vi "SetMode.vi"(0 "VISA resource name":refnum<visa-resource-name>, 5 "Combo Box":string(combo), 11 "error in (no error)":errorcluster) -> (4 "VISA resource name out":refnum<visa-resource-name>, 15 "error out":errorcluster)   [LabVIEW 2024, in "EFmeter.lvlib"]
uses:
  EFmeter.lvlib
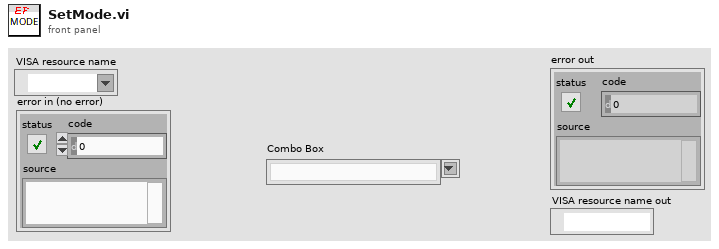
[diagram p1: front panel]
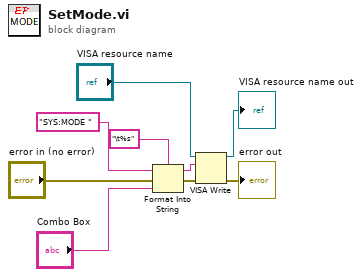
[diagram p0: block diagram]
diagram:
  n1 = Format Into String(format string="\t%s", initial string="SYS:MODE ", error in="error in (no error)", "Combo Box") -> (resulting string=w1:string, error out=w7:errorcluster)
  n2 = VISA Write(VISA resource name="VISA resource name", write buffer=w1, error in (no error)=w7) -> (VISA resource name out=→"VISA resource name out":refnum<visa-resource-name>, error out=→"error out":errorcluster)  [unwired: 1 out]
